vi "RunningAverage.vi"(2 "New Value":u64, 3 "Fixed Size Array\nOf Previous Values":u64[](array[numeric])) -> (0 "Average Value":dbl, 1 "New Fixed Size Array":u64[](array[numeric]))   [LabVIEW 2016]
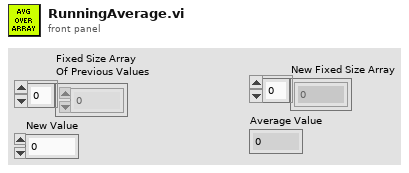
[diagram p1: front panel]
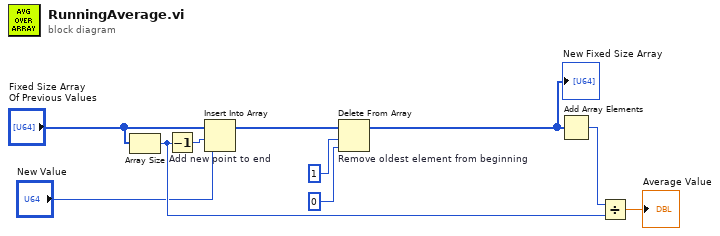
[diagram p0: block diagram]
diagram:
  n1 = Array Size(array="Fixed Size Array\nOf Previous Values") -> (size(s)=w2:i32)
  n2 = Decrement(x=w2) -> (x-1=w5:i32)
  n3 = Insert Into Array "Add new point to end"(array="Fixed Size Array\nOf Previous Values", index=w5, new element="New Value") -> (w10:u64[])
  n4 = Delete From Array "Remove oldest element from beginning"(array=w10, length=1, index=0) -> (array with subset deleted=w7:u64[])  [unwired: 1 out]
  "New Fixed Size Array" <- w7
  n5 = Add Array Elements(numeric array=w7) -> (sum=w6:u64)
  n6 = Divide(x=w6, y=w2) -> (x/y=→"Average Value":dbl)
